vi "Teardown.vi"(7 "Actor in":refnum<class "Actor.lvclass">, 11 "Destroy State in":refnum<class "Destroy State.lvclass">) -> (2 "Teardown?":bool, 5 "Actor out":refnum<class "Actor.lvclass">)   [LabVIEW 2021, in "jettl.lvlib" / "Destroy State.lvclass"]
uses:
  Destroy State.lvclass
  Actor/Actor/Actor.lvclass
  Actor/Msgs/Last Ack/Last Ack Msg/Last Ack Msg.lvclass
  C:/git/jettl/src/Actor/Msg/Msg.lvclass
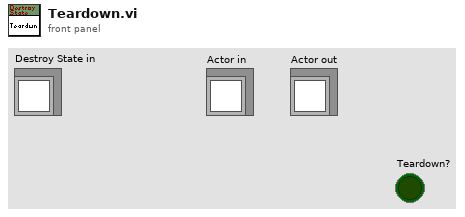
[diagram p1: front panel]
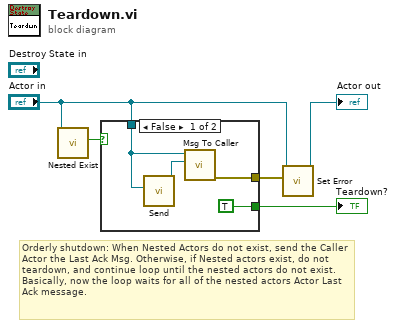
[diagram p0: block diagram]
diagram:
  # "Orderly shutdown: When Nested Actors do not exist, send the Caller Actor the Last Ack Msg. Otherwise, if Nested actors exist, do not teardown, and continue loop until the nested actors do not exist. Basically, now the loop waits for all of the nested actors Actor Last Ack message."
  n1 = call-dynamic "Nested Exist.vi"("Actor in"="Actor in") -> ("Nested Exist?"=w4:bool)  [unwired: 10 in]
  n2 = case shown="False" w4 {
    tunnel: "Actor in" -> [w8 _]
    tunnel: [TRUE ("Destroyed?") _] -> w5
    tunnel: [w6 _] -> w2
    frame False {
      n3 = call "Send.vi"("Actor"=w8) -> ("Last Ack Msg out"=w7:refnum<class "Last Ack Msg.lvclass">)  [unwired: 10 in]
      n4 = call-dynamic "Msg To Caller.vi"("Msg"=w7, "Actor in"=w8) -> ("error out"=w6:errorcluster)  [unwired: 9 in]
    }
    frame True {
    }
  }
  "Teardown?" <- w5
  n5 = call-dynamic "Set Error.vi"("Merge"=w2, "Set Error in"="Actor in") -> ("Set Error out"=→"Actor out":refnum<class "Actor.lvclass">)  [unwired: 9 in]
